vi "AddGlyphtoGManager.vi"(8 "error in":errorcluster, 10 "glyph manager":T1, 11 "CVT Engine Editor in":refnum<class "CVT Engine Editor.lvclass">) -> (0 "error out":errorcluster, 2 "glyph manager out":T1, 3 "CVT Engine Editor out":refnum<class "CVT Engine Editor.lvclass">)   [LabVIEW 2013, in "CVT Engine Editor.lvclass"]
uses:
  CVT Engine Editor.lvclass
  <vilib>/NI/Configuration Framework/glyph manager/glyph manager.ctl
  <vilib>/picture/picture.llb/imagedata.ctl
  <vilib>/NI/Tag Bus Data Framework/Configuration Editor/Classes/Engine Parent/Engine Parent Editor Node.lvclass
  <vilib>/NI/Configuration Framework/glyph manager/glyph manager.lvlib
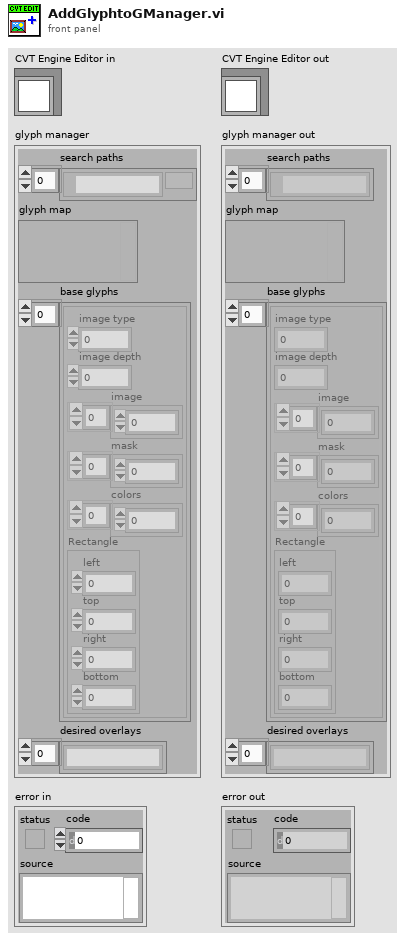
[diagram p1: front panel]
types:
  T1 = typedef "glyph manager.lvlib/glyph manager.ctl" = cluster{"search paths":path[], "glyph map":variant, "base glyphs":T2[], "desired overlays":string[]}
  T2 = typedef "imagedata.ctl" = cluster{"image type":i32, "image depth":i32, "image":u8[], "mask":u8[], "colors":u32[], "Rectangle":cluster{"left":i16, "top":i16, "right":i16, "bottom":i16}}
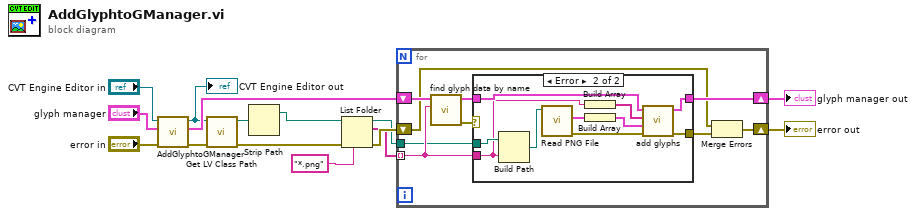
[diagram p0: block diagram]
diagram:
  n1 = call-parent "AddGlyphtoGManager.vi"("error in"="error in", "glyph manager"="glyph manager", "NISE_CEF_serializable node in"="CVT Engine Editor in") -> ("error out"=w4:errorcluster, "glyph manager out"=w6:T1, "NISE_CEF_serializable node out"=w2:refnum<class "CVT Engine Editor.lvclass">)  [unwired: 6 in]
  "CVT Engine Editor out" <- w2
  n2 = call <vilib>:"Get LV Class Path.vi"("error in (no error)"=w4, "object"=w2) -> ("error out"=w10:errorcluster, "class path"=w9:path)  [unwired: 8 in]
  n3 = Strip Path(path=w9) -> (stripped path=w11:path)  [unwired: 1 out]
  n4 = List Folder(path=w11, pattern="*.png", error in=w10) -> (path out=w1:path, filenames=w3:string[], error out=w5:errorcluster)  [unwired: 1 in, 1 out]
  n5 = for {
    tunnel: w3 -> [w19] mode=indexing
    shift-right: [w22] -> w14
    shift-left: w6 -> [w20]
    shift-right: [w18] -> w13
    shift-left: w5 -> [w17]
    tunnel: w1 -> [w16]
    n6 = call <vilib>:"find glyph data by name.vi"("name"=w19, "glyph manager in"=w20) -> ("error out"=w24:errorcluster, "glyph manager out"=w23:T1)  [unwired: 6 in, 2 out]
    n7 = case shown="Error" w24 {
      selector: w24 -> [w26 _]
      tunnel: [w26 w35] -> w21
      tunnel: w23 -> [w25 w33]
      tunnel: [w25 w34] -> w22
      tunnel: w19 -> [_ w28]
      tunnel: w16 -> [_ w30]
      frame No Error {
      }
      frame Error {
        n8 = Build Path(base path=w30, name or relative path=w28) -> (appended path=w27:path)
        n9 = call <vilib>:"Read PNG File.vi"("path to PNG file"=w27) -> ("error out"=w36:errorcluster, "image data"=w29:T2)  [unwired: 8 in, 1 out]
        n10 = Build Array(w28) -> (w32:string[])
        n11 = Build Array(w29) -> (w31:T2[])
        n12 = call <vilib>:"add glyphs.vi"("error in"=w36, "glyphs"=w31, "names"=w32, "glyph manager in"=w33) -> ("error out"=w35:errorcluster, "glyph manager out"=w34:T1)  [unwired: 6 in]
      }
    }
    n13 = Merge Errors(w17, w21) -> (w18:errorcluster)
  }
  "error out" <- w13
  "glyph manager out" <- w14
